vi "setup complete.vi"() -> ()   [LabVIEW 2014]
uses:
  <vilib>/Utility/sysdir.llb/System Directory Type.ctl
panel:
  in  "?":bool
  out "메시지":string
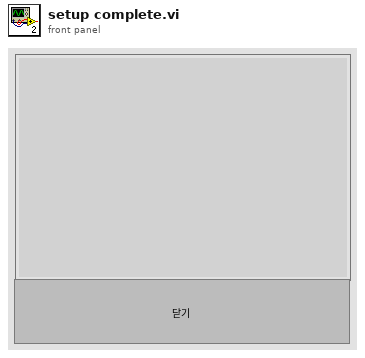
[diagram p1: front panel]
types:
  T1 = typedef "System Directory Type.ctl" = i32
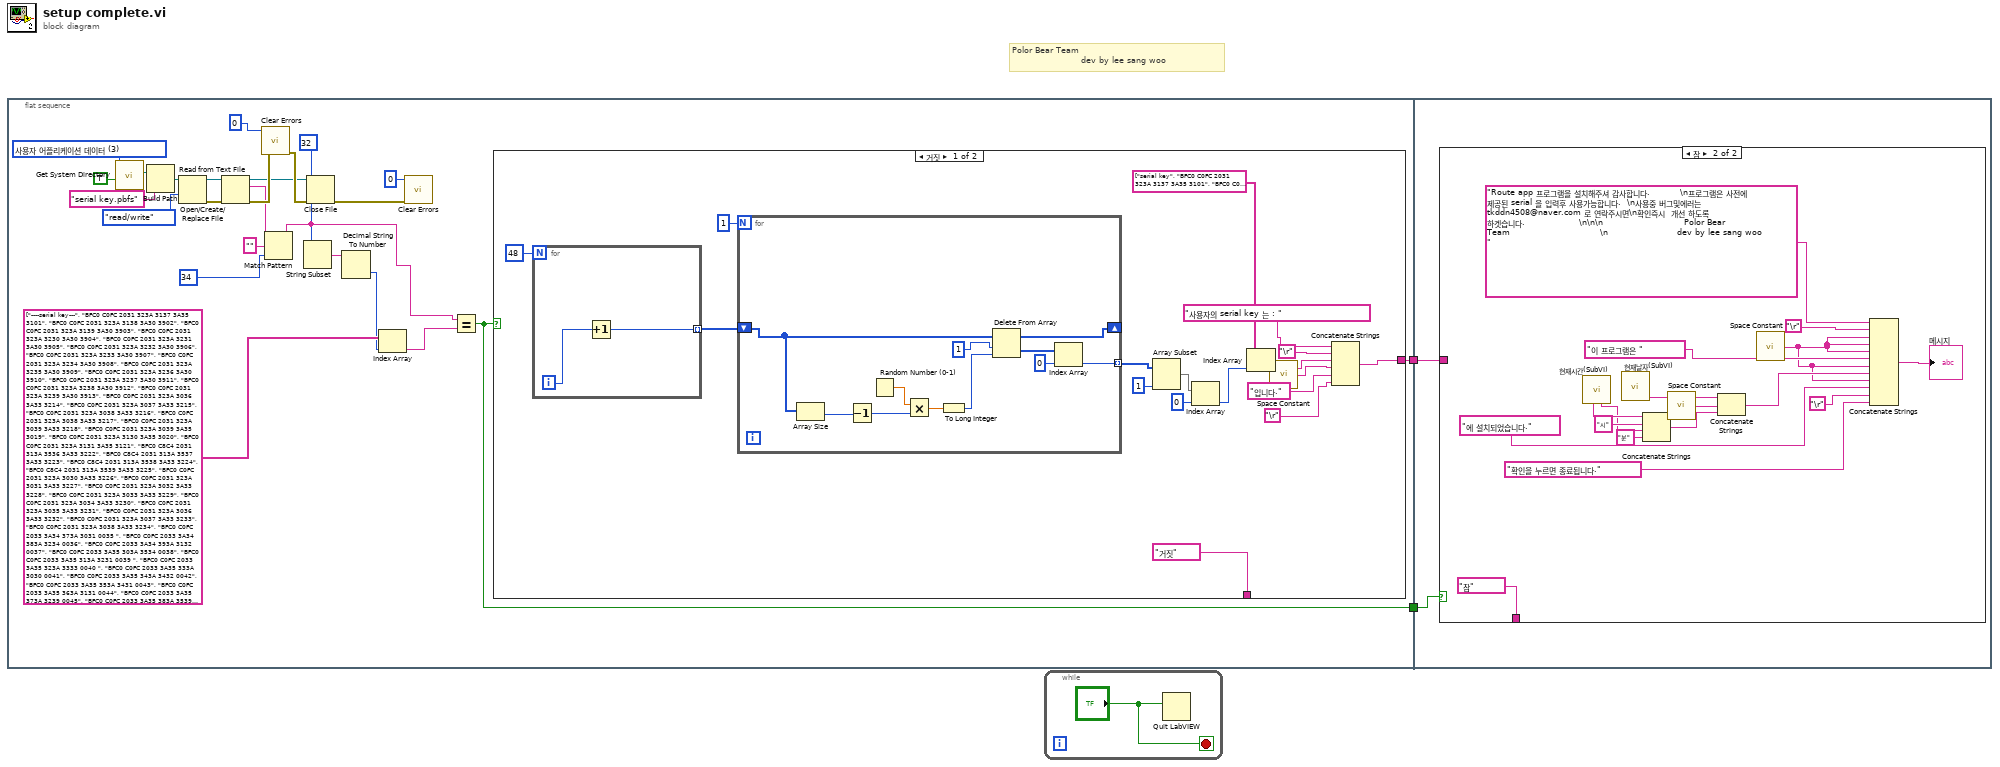
[diagram p0: block diagram]
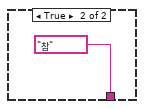
[diagram p2: hidden frame]
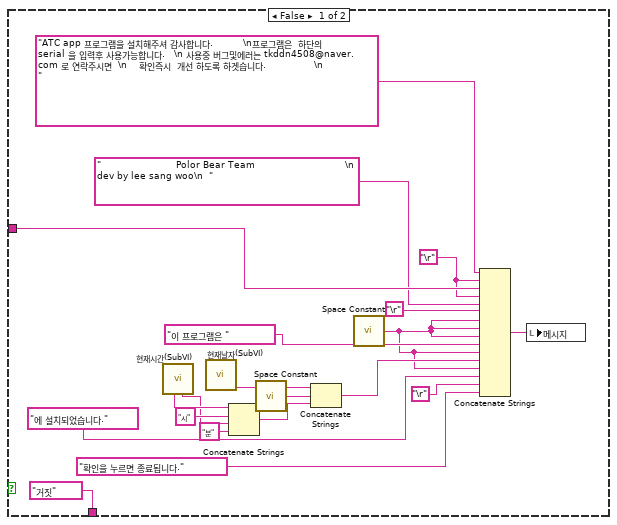
[diagram p3: hidden frame]
diagram:
  # "Polor Bear Team                              \n                       dev by lee sang woo"
  n1 = flat-sequence {
    tunnel: [w7] -> w2
    tunnel: [w6] -> w1
    tunnel: w2 -> [w60]
    tunnel: w1 -> [w59]
    frame #0 {
      w22 = T1 3 items=["사용자 홈"=0, "사용자 데스크탑"=1, "사용자 문서"=2, "사용자 어플리케이션 데이터"=3, "사용자 환경"=4, "사용자 임시"=5, "퍼블릭 문서"=6, "퍼블릭 어플리케이션 데이터"=7, "퍼블릭 환경"=8, "퍼블릭 캐시"=13, "시스템 코어 라이브러리"=9, "시스템 설치된 라이브러리"=10, "어플리케이션 파일"=11, "부팅 볼륨 루트"=12] ("system directory type")
      n2 = call <vilib>:"Get System Directory.vi"("create directory if not found? (F)"=TRUE, "system directory type"=w22) -> ("system directory"=w23:path)  [unwired: 9 in]
      n3 = Build Path(base path=w23, name or relative path="serial key.pbfs" ("이름 또는 상대 경로")) -> (appended path=w24:path)
      n4 = Open/Create/Replace File(file path (use dialog)=w24, access (0:read/write)=enum16{"read/write", "read-only", "write-only"}."read/write" ("접근(0:읽기/쓰기)")) -> (refnum out=w18:refnum<file>, error out=w19:errorcluster)  [unwired: 4 in, 1 out]
      n5 = Read from Text File(file (use dialog)=w18, error in=w19) -> (refnum out=w17:refnum<file>, text=w9:string, error out=w25:errorcluster)  [unwired: 2 in, 1 out]
      n6 = call <vilib>:"Clear Errors.vi"("error in (no error)"=w25, "specific error code to clear (0: all)"=0) -> ("error out"=w26:errorcluster)  [unwired: 4 in, 1 out]
      n7 = Match Pattern(string=w9, regular expression="" ("정규식"), offset (0)=34 ("오프셋(0)")) -> (before substring=w3:string)  [unwired: 3 out]
      n8 = String Subset(string=w3, offset (0)=32 ("오프셋(0) 2")) -> (substring=w13:string)  [unwired: 1 in]
      n9 = Close File(refnum=w17, error in=w26) -> (error out=w5:errorcluster)  [unwired: 1 out]
      n10 = Decimal String To Number(string=w13) -> (number=w10:i32)  [unwired: 2 in, 1 out]
      n11 = Index Array(array=string[] ["----serial key---", "BFC0 C0FC 2031 323A 3137 3A35 3101", "BFC0 C0FC 2031 323A 3138 3A30 3902", "BFC0 C0FC 2031 323A 3139 3A30 3903", "BFC0 C0FC 2031 323A 3230 3A30 3904", "BFC0 C0FC 2031 323A 3231 3A30 3905", "BFC0 C0FC 2031 323A 3232 3A30 3906", "BFC0 C0FC 2031 323A 3233 3A30 3907", "BFC0 C0FC 2031 323A 3234 3A30 3908", "BFC0 C0FC 2031 323A 3235 3A30 3909", "BFC0 C0FC 2031 323A 3236 3A30 3910", "BFC0 C0FC 2031 323A 3237 3A30 3911", "BFC0 C0FC 2031 323A 3238 3A30 3912", "BFC0 C0FC 2031 323A 3239 3A30 3913", "BFC0 C0FC 2031 323A 3036 3A33 3214", "BFC0 C0FC 2031 323A 3037 3A33 3215", "BFC0 C0FC 2031 323A 3038 3A33 3216", "BFC0 C0FC 2031 323A 3038 3A33 3217", "BFC0 C0FC 2031 323A 3039 3A33 3218", "BFC0 C0FC 2031 323A 3039 3A35 3019", "BFC0 C0FC 2031 323A 3130 3A35 3020", "BFC0 C0FC 2031 323A 3131 3A35 3121", "BFC0 C8C4 2031 313A 3536 3A33 3222", "BFC0 C8C4 2031 313A 3537 3A33 3223", "BFC0 C8C4 2031 313A 3538 3A33 3224", "BFC0 C8C4 2031 313A 3539 3A33 3225", "BFC0 C0FC 2031 323A 3030 3A33 3226", "BFC0 C0FC 2031 323A 3031 3A33 3227", "BFC0 C0FC 2031 323A 3032 3A33 3228", "BFC0 C0FC 2031 323A 3033 3A33 3229", "BFC0 C0FC 2031 323A 3034 3A33 3230", "BFC0 C0FC 2031 323A 3035 3A33 3231", "BFC0 C0FC 2031 323A 3036 3A33 3232", "BFC0 C0FC 2031 323A 3037 3A33 3233", "BFC0 C0FC 2031 323A 3038 3A33 3234", "BFC0 C0FC 2033 3A34 373A 3031 0035 ", "BFC0 C0FC 2033 3A34 383A 3234 0036", "BFC0 C0FC 2033 3A34 393A 3132 0037", "BFC0 C0FC 2033 3A35 303A 3534 0038", "BFC0 C0FC 2033 3A35 313A 3231 0039 ", "BFC0 C0FC 2033 3A35 323A 3333 0040 ", "BFC0 C0FC 2033 3A35 333A 3030 0041", "BFC0 C0FC 2033 3A35 343A 3432 0042", "BFC0 C0FC 2033 3A35 353A 3431 0043", "BFC0 C0FC 2033 3A35 363A 3131 0044", "BFC0 C0FC 2033 3A35 373A 3239 0045", "BFC0 C0FC 2033 3A35 383A 3539 0046", "BFC0 C0FC 2033 3A35 393A 3533 0047", "BFC0 C0FC 2034 3A30 303A 3430 0048 "] ("출력 배열"), index=w10) -> (element=w8:string)
      n12 = call <vilib>:"Clear Errors.vi"("error in (no error)"=w5, "specific error code to clear (0: all)"=0) -> ()  [unwired: 4 in, 2 out]
      n13 = Equal?(x=w3, y=w8) -> (x = y?=w7:bool)
      n14 = case shown="거짓" w7 {
        tunnel: [w32 _] -> w6
        tunnel: ["거짓" "참"] -> _
        frame False {
          n15 = for {
            N: 48 -> [_]
            tunnel: [w56] -> w43 mode=indexing
            i -> [w57]
            n16 = Increment(x=w57) -> (x+1=w56:i32)
          }
          n17 = for {
            N: 1 -> [_]
            shift-right: [w55] -> _
            shift-left: w43 -> [w50]
            tunnel: [w45] -> w42 mode=indexing
            n18 = Array Size(array=w50) -> (size(s)=w51:i32)
            n19 = Decrement(x=w51) -> (x-1=w49:i32)
            n20 = Random Number (0-1)() -> (number: 0 to 1=w52:dbl)
            n21 = Multiply(x=w52, y=w49) -> (x*y=w48:dbl)
            n22 = To Long Integer(number=w48) -> (32bit integer=w47:i32)
            n23 = Delete From Array(array=w50, length=1, index=w47) -> (deleted portion=w46:i32[], array with subset deleted=w55:i32[])
            n24 = Index Array(array=w46, index=0 ("인덱스")) -> (element=w45:i32)
          }
          n25 = Array Subset(array=w42, length=1 ("길이")) -> (w39:i32[])  [unwired: 1 in]
          n26 = Index Array(array=w39, index=0 ("인덱스")) -> (element=w37:i32)
          n27 = Index Array(array=string[] ["serial key", "BFC0 C0FC 2031 323A 3137 3A35 3101", "BFC0 C0FC 2031 323A 3138 3A30 3902", "BFC0 C0FC 2031 323A 3139 3A30 3903", "BFC0 C0FC 2031 323A 3230 3A30 3904", "BFC0 C0FC 2031 323A 3231 3A30 3905", "BFC0 C0FC 2031 323A 3232 3A30 3906", "BFC0 C0FC 2031 323A 3233 3A30 3907", "BFC0 C0FC 2031 323A 3234 3A30 3908", "BFC0 C0FC 2031 323A 3235 3A30 3909", "BFC0 C0FC 2031 323A 3236 3A30 3910", "BFC0 C0FC 2031 323A 3237 3A30 3911", "BFC0 C0FC 2031 323A 3238 3A30 3912", "BFC0 C0FC 2031 323A 3239 3A30 3913", "BFC0 C0FC 2031 323A 3036 3A33 3214", "BFC0 C0FC 2031 323A 3037 3A33 3215", "BFC0 C0FC 2031 323A 3038 3A33 3216", "BFC0 C0FC 2031 323A 3038 3A33 3217", "BFC0 C0FC 2031 323A 3039 3A33 3218", "BFC0 C0FC 2031 323A 3039 3A35 3019", "BFC0 C0FC 2031 323A 3130 3A35 3020", "BFC0 C0FC 2031 323A 3131 3A35 3121", "BFC0 C8C4 2031 313A 3536 3A33 3222", "BFC0 C8C4 2031 313A 3537 3A33 3223", "BFC0 C8C4 2031 313A 3538 3A33 3224", "BFC0 C8C4 2031 313A 3539 3A33 3225", "BFC0 C0FC 2031 323A 3030 3A33 3226", "BFC0 C0FC 2031 323A 3031 3A33 3227", "BFC0 C0FC 2031 323A 3032 3A33 3228", "BFC0 C0FC 2031 323A 3033 3A33 3229", "BFC0 C0FC 2031 323A 3034 3A33 3230", "BFC0 C0FC 2031 323A 3035 3A33 3231", "BFC0 C0FC 2031 323A 3036 3A33 3232", "BFC0 C0FC 2031 323A 3037 3A33 3233", "BFC0 C0FC 2031 323A 3038 3A33 3234", "BFC0 C0FC 2033 3A34 373A 3031 0035 ", "BFC0 C0FC 2033 3A34 383A 3234 0036", "BFC0 C0FC 2033 3A34 393A 3132 0037", "BFC0 C0FC 2033 3A35 303A 3534 0038", "BFC0 C0FC 2033 3A35 313A 3231 0039 ", "BFC0 C0FC 2033 3A35 323A 3333 0040 ", "BFC0 C0FC 2033 3A35 333A 3030 0041", "BFC0 C0FC 2033 3A35 343A 3432 0042", "BFC0 C0FC 2033 3A35 353A 3431 0043", "BFC0 C0FC 2033 3A35 363A 3131 0044", "BFC0 C0FC 2033 3A35 373A 3239 0045", "BFC0 C0FC 2033 3A35 383A 3539 0046", "BFC0 C0FC 2033 3A35 393A 3533 0047", "BFC0 C0FC 2034 3A30 303A 3430 0048 "] ("출력 배열"), index=w37) -> (element=w34:string)
          n28 = call <vilib>:"Space Constant.vi"() -> ("String"=w31:string)
          n29 = Concatenate Strings("사용자의 serial key 는 : " ("문자열"), "\r", w34, w31, "입니다." ("문자열"), "\r") -> (w32:string)
        }
        frame True {
        }
      }
    }
    frame #1 {
      n30 = case shown="참" w60 {
        tunnel: w59 -> [w64 _]
        tunnel: ["거짓" "참"] -> _
        frame False {
          w63 = "\r"
          n31 = call "현재시간(SubVI).vi"() -> ("분 문자열"=w78:string, "시 문자열"=w80:string)  [unwired: 3 in, 7 out]
          n32 = call "현재날자(SubVI).vi"() -> ("월,일 을 문자열로"=w74:string)  [unwired: 5 in, 6 out]
          n33 = Concatenate Strings(w80, "시", w78, "분" ("문자열")) -> (w76:string)
          n34 = call <vilib>:"Space Constant.vi"() -> ("String"=w75:string)
          n35 = Concatenate Strings(w74, w75, w76) -> (w71:string)
          n36 = call <vilib>:"Space Constant.vi"() -> ("String"=w70:string)
          n37 = Concatenate Strings("ATC app 프로그램을 설치해주셔 감사합니다.          \n프로그램은  하단의  serial 을 입력후 사용가능합니다.   \n 사용중 버그및에러는 tkddn4508@naver.com 로 연락주시면  \n    확인즉시  개선 하도록 하겟습니다.                \n                                       " ("Message"), w63, w64, w63, "                         Polor Bear Team                              \n                       dev by lee sang woo\n  ", "\r", w70, w70, w70, "이 프로그램은 ", w70, w71, w70, "에 설치되었습니다.", "\r", "확인을 누르면 종료됩니다.") -> (w66:string)
          n38 = local write "메시지"(w66) -> ()
        }
        frame True {
          n39 = call "현재시간(SubVI).vi"() -> ("분 문자열"=w95:string, "시 문자열"=w97:string)  [unwired: 3 in, 7 out]
          n40 = call "현재날자(SubVI).vi"() -> ("월,일 을 문자열로"=w91:string)  [unwired: 5 in, 6 out]
          n41 = Concatenate Strings(w97, "시", w95, "분" ("문자열")) -> (w93:string)
          n42 = call <vilib>:"Space Constant.vi"() -> ("String"=w92:string)
          n43 = Concatenate Strings(w91, w92, w93) -> (w87:string)
          n44 = call <vilib>:"Space Constant.vi"() -> ("String"=w86:string)
          n45 = Concatenate Strings("Route app 프로그램을 설치해주셔 감사합니다.          \n프로그램은 사전에 제공된 serial 을 입력후 사용가능합니다.  \n사용중 버그및에러는 tkddn4508@naver.com 로 연락주시면\n확인즉시  개선 하도록 하겟습니다.                  \n\n\n                           Polor Bear Team                              \n                       dev by lee sang woo                            " ("Message"), "\r", w86, w86, w86, "이 프로그램은 ", w86, w87, w86, "에 설치되었습니다.", "\r", "확인을 누르면 종료됩니다.") -> (→"메시지":string)
        }
      }
    }
  }
  n46 = while {
    stop <- "?" stop-if-true
    n47 = Quit LabVIEW(quit? (T)="?") -> ()
  }
